vi "conversion.vi"() -> ()   [LabVIEW 2017]
uses:
  test_section_physical_channels.ctl
panel:
  in  "cluster 2":T1
  out "cluster":T2
  out "Numeric":i32
  out "Type":string[](array[string])
  out "Module":string[](array[string])
  out "Channel":string[](array[string])
  out "Name":string[](array[string])
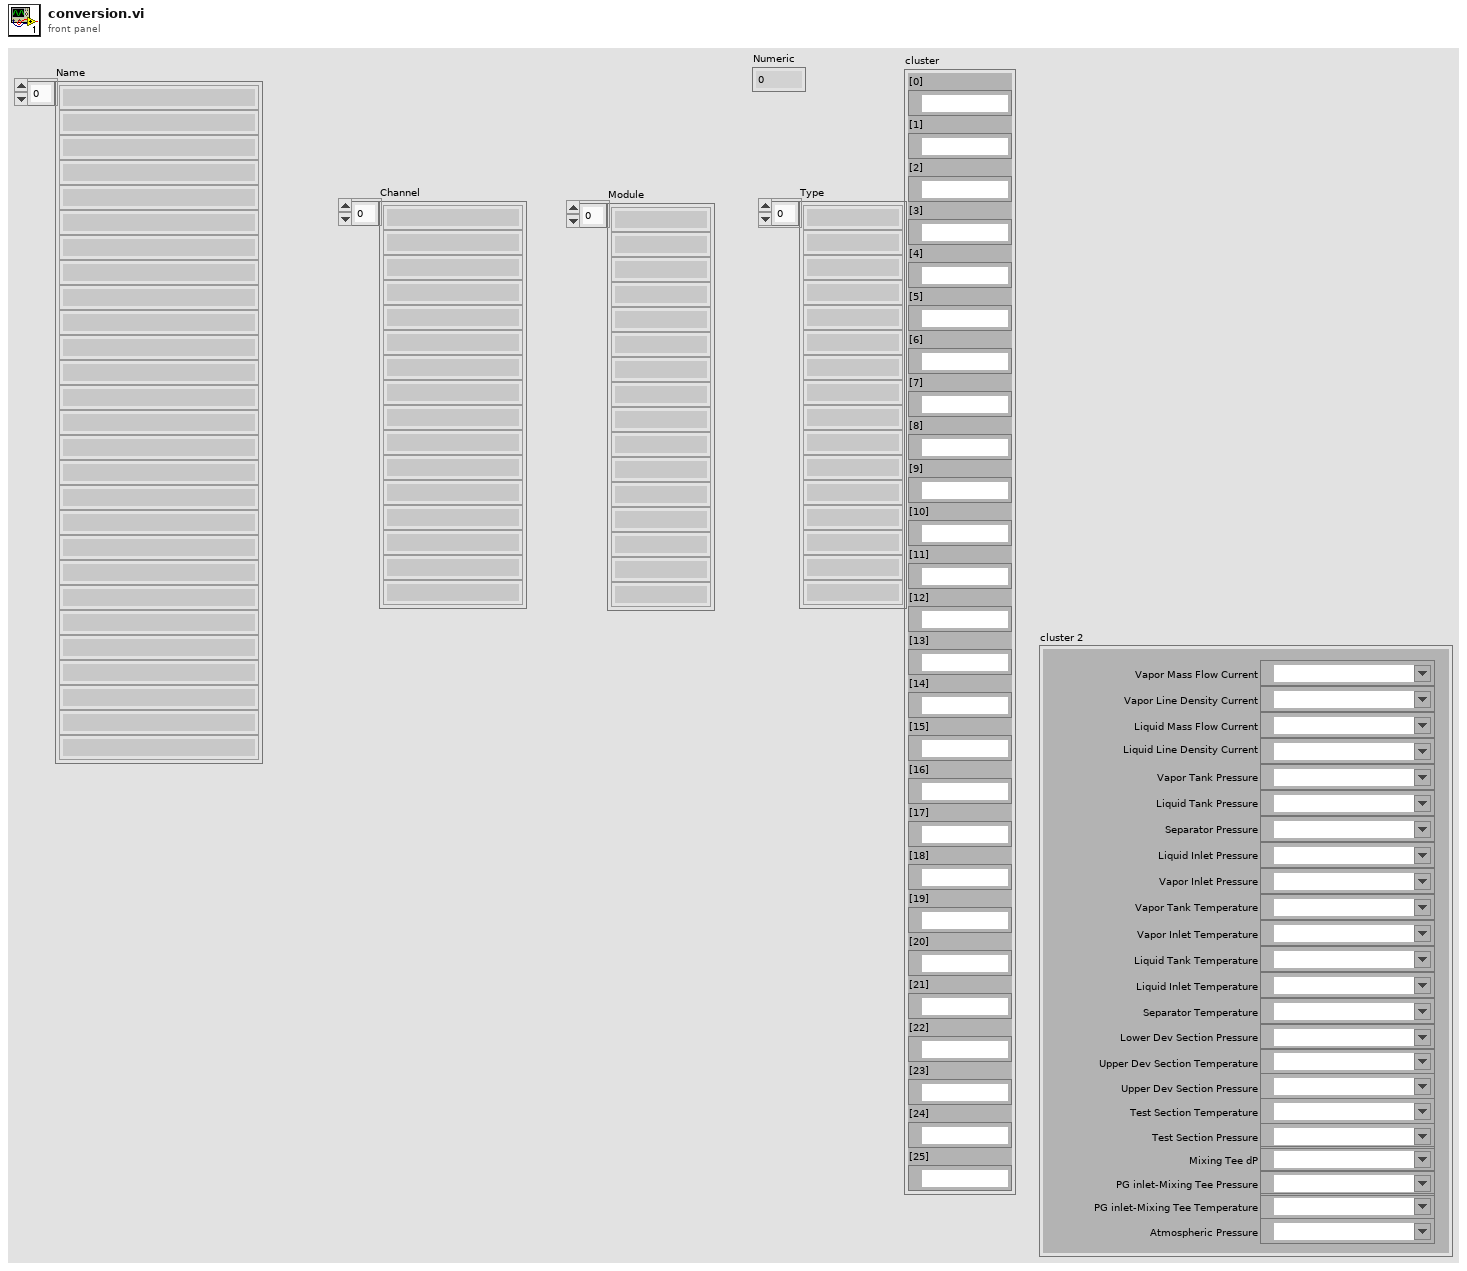
[diagram p1: front panel]
types:
  T1 = typedef "test_section_physical_channels.ctl" = cluster{"Vapor Mass Flow Current":tag, "Vapor Line Density Current":tag, "Liquid Mass Flow Current":tag, "Liquid Line Density Current":tag, "Vapor Tank Pressure":tag, "Liquid Tank Pressure":tag, "Separator Pressure":tag, "Liquid Inlet Pressure":tag, "Vapor Inlet Pressure":tag, "Vapor Tank Temperature":tag, "Vapor Inlet Temperature":tag, "Liquid Tank Temperature":tag, "Liquid Inlet Temperature":tag, "Separator Temperature":tag, "Lower Dev Section Pressure":tag, "Test Section Temperature":tag, "Upper Dev Section Temperature":tag, "Upper Dev Section Pressure":tag, "Atmospheric Pressure":tag, "Mixing Tee dP":tag, "PG inlet-Mixing Tee Pressure":tag, "Test Section Pressure":tag, "PG inlet-Mixing Tee Temperature":tag}
  T2 = cluster{"[0]":tag, "[1]":tag, "[2]":tag, "[3]":tag, "[4]":tag, "[5]":tag, "[6]":tag, "[7]":tag, "[8]":tag, "[9]":tag, "[10]":tag, "[11]":tag, "[12]":tag, "[13]":tag, "[14]":tag, "[15]":tag, "[16]":tag, "[17]":tag, "[18]":tag, "[19]":tag, "[20]":tag, "[21]":tag, "[22]":tag, "[23]":tag, "[24]":tag, "[25]":tag}
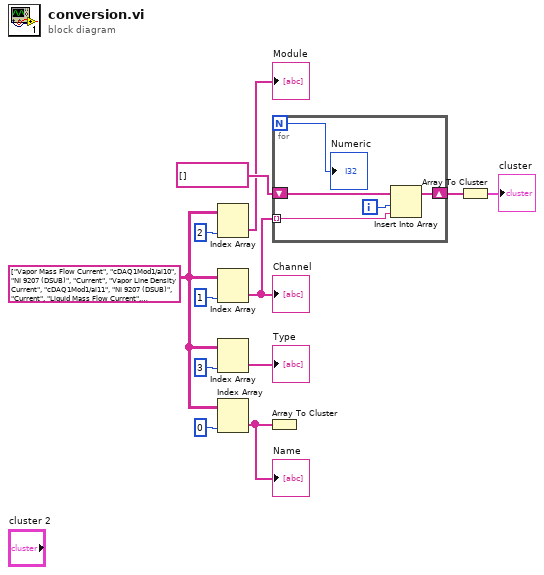
[diagram p0: block diagram]
diagram:
  w4 = string[][] [["Vapor Mass Flow Current", "cDAQ1Mod1/ai10", "NI 9207 (DSUB)", "Current"], ["Vapor Line Density Current", "cDAQ1Mod1/ai11", "NI 9207 (DSUB)", "Current"], ["Liquid Mass Flow Current", "cDAQ1Mod1/ai8", "NI 9207 (DSUB)", "Current"], ["Liquid Line Density Current", "cDAQ1Mod1/ai9", "NI 9207 (DSUB)", "Current"], ["Vapor Tank Pressure", "cDAQ1Mod1/ai3", "NI 9207 (DSUB)", "Voltage"], ["Liquid Tank Pressure", "cDAQ1Mod1/ai2", "NI 9207 (DSUB)", "Voltage"], ["Separator Pressure", "cDAQ1Mod1/ai4", "NI 9207 (DSUB)", "Voltage"], ["Liquid Inlet Pressure", "cDAQ1Mod1/ai0", "NI 9207 (DSUB)", "Voltage"], ["Dev Section Pressure", "cDAQ1Mod1/ai1", "NI 9207 (DSUB)", "Voltage"], ["Vapor Tank Temp", "cDAQ1Mod6/ai2", "NI 9213", "Thermocouple"], ["Vapor Inlet Temp", "cDAQ1Mod6/ai0", "NI 9213", "Thermocouple"], ["Liquid Tank Temp", "cDAQ1Mod6/ai3", "NI 9213", "Thermocouple"], ["Liquid Inlet Temp", "cDAQ1Mod6/ai4", "NI 9213", "Thermocouple"], ["Separator Temp", "cDAQ1Mod6/ai1", "NI 9213", "Thermocouple"], ["Lower Test Section Pressure", "cDAQ1Mod1/ai5", "NI 9207 (DSUB)", "Voltage"], ["Lower Test Section Temp", "cDAQ1Mod6/ai5", "NI 9213", "Thermocouple"], ["Top Heater Temp", "cDAQ1Mod6/ai6", "NI 9213", "Voltage"], ["Bottom Heater Temp", "cDAQ1Mod6/ai7", "NI 9213", "Voltage"], ["Pressure Drop", "cDAQ1Mod1/ai12", "NI 9207 (DSUB)", "Current"], ["Upper test section Temp", "cDAQ1Mod6/ai9", "NI 9213", "Thermocouple"], ["Upper TS Pressure", "cDAQ1Mod1/ai7", "NI 9207 (DSUB)", "Voltage"], ["Condenser Top Temp", "cDAQ1Mod6/ai8", "NI 9213", "Voltage"], ["Condenser Bottom Temp", "cDAQ1Mod6/ai10", "NI 9213", "Voltage"], ["Evaporator top temp", "cDAQ1Mod6/ai11", "NI 9213", "Thermocouple"], ["Evaporator Bottom Temp", "cDAQ1Mod6/ai12", "NI 9213", "Voltage"], ["Test Section Window 3-4 P", "cDAQ1Mod1/ai6", "NI 9207 (DSUB)", "Voltage"]] ("all rows 2")
  n1 = Index Array(array=w4, index (col)=2 ("index")) -> (element=→"Module":string[])  [unwired: 1 in]
  n2 = Index Array(array=w4, index (col)=1 ("index")) -> (element=w5:string[])  [unwired: 1 in]
  "Channel" <- w5
  n3 = Index Array(array=w4, index (col)=3 ("index")) -> (element=→"Type":string[])  [unwired: 1 in]
  n4 = Index Array(array=w4, index (col)=0 ("index")) -> (element=w3:string[])  [unwired: 1 in]
  "Name" <- w3
  n5 = Array To Cluster(array=w3) -> ()  [unwired: 1 out]
  n6 = for {
    N -> [w13]
    tunnel: w5 -> [w16] mode=indexing
    shift-right: [w15] -> w2
    shift-left: tag[] [] -> [w17]
    i -> [w14]
    n7 = Insert Into Array(array=w17, index=w14, new element=w16) -> (w15:tag[])
    "Numeric" <- w13
  }
  n8 = Array To Cluster(array=w2) -> (cluster=→"cluster":T2)
